vi "MAT.vi"(8 "Alfa term":dbl, 10 "Current":dbl[](array[numeric]), 11 "Voltage":dbl[](array[numeric])) -> (0 "u_A":dbl, 1 "avg_temp":dbl, 2 "Resistance":dbl[](array[numeric]), 3 "Temp":dbl[](array[numeric]))   [LabVIEW 2022 SP3]
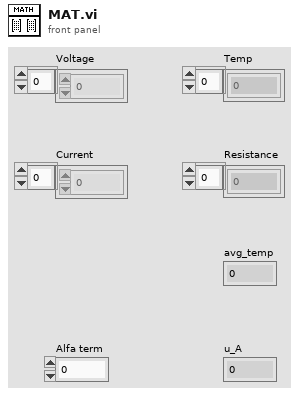
[diagram p1: front panel]
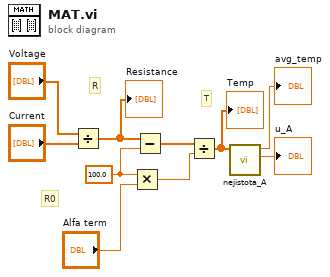
[diagram p0: block diagram]
diagram:
  w8 = 100.0 ("Numeric")
  # "T"
  # "R0"
  # "R"
  n1 = Divide(x="Voltage", y="Current") -> (x/y=w2:dbl[])
  "Resistance" <- w2
  n2 = Multiply(x=w8, y="Alfa term") -> (x*y=w5:dbl)
  n3 = Subtract(x=w2, y=w8) -> (x-y=w6:dbl[])
  n4 = Divide(x=w6, y=w5) -> (x/y=w1:dbl[])
  "Temp" <- w1
  n5 = call "nejistota_A.vi"("Array"=w1) -> ("nejistota_A"=→"u_A":dbl, "mean"=→"avg_temp":dbl)  [unwired: 9 in]
